vi "Is function supported.vi"(8 "error in (no error)":errorcluster, 10 "Hardware function":T1, 11 "Mag Lab Hardware in":refnum<class "Mag Lab Hardware.lvclass">) -> (0 "error out":errorcluster, 2 "Supported":bool, 3 "Mag Lab Hardware out":refnum<class "Mag Lab Hardware.lvclass">)   [LabVIEW 2015, in "Mag Lab Hardware.lvclass"]
uses:
  Mag Lab Hardware.lvclass
  Mag Lab Hardware Function.ctl
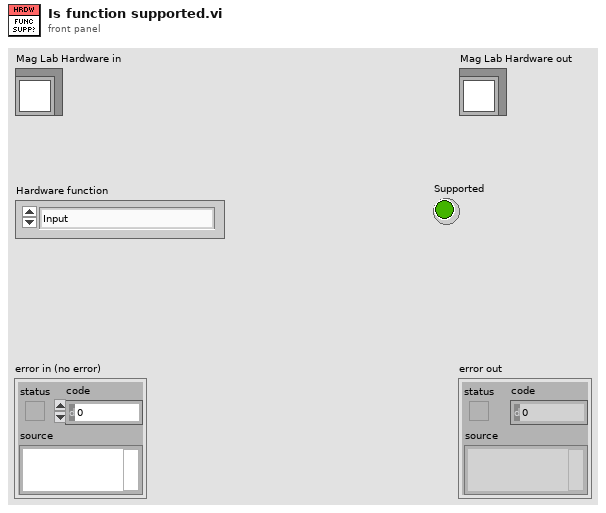
[diagram p1: front panel]
types:
  T1 = typedef "Mag Lab Hardware Function.ctl" = enum16{"Input", "Voltmeter", "Output", "Current source", "Digitizer", "Temperature controller"}
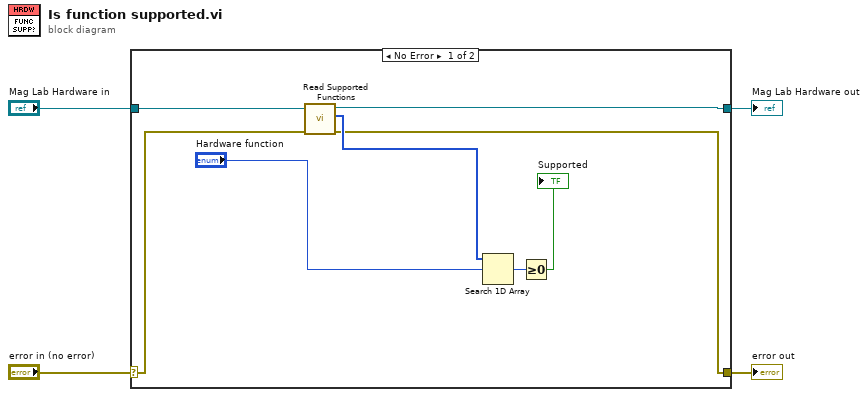
[diagram p0: block diagram]
diagram:
  n1 = case shown="No Error" "error in (no error)" {
    selector: "error in (no error)" -> [w5 w14]
    tunnel: [w6 w14] -> w3
    tunnel: [w7 w13] -> w1
    tunnel: "Mag Lab Hardware in" -> [w12 w13]
    frame No Error {
      n2 = call-dynamic "Read Supported Functions.vi"("error in (no error)"=w5, "Mag Lab Hardware in"=w12) -> ("error out"=w6:errorcluster, "Supported Functions"=w11:T1[], "Mag Lab Hardware out"=w7:refnum<class "Mag Lab Hardware.lvclass">)  [unwired: 7 in]
      n3 = Search 1D Array(1D array=w11, element="Hardware function") -> (index of element=w9:i32)  [unwired: 1 in]
      n4 = Greater Or Equal To 0?(x=w9) -> (x >= 0?=→"Supported":bool)
    }
    frame Error {
    }
  }
  "error out" <- w3
  "Mag Lab Hardware out" <- w1
